vi "test_Are All Channels Defined.vi"(8 "error in":errorcluster) -> (0 "error out":errorcluster)   [LabVIEW 2020, in "Test_Routing Templates.lvlib"]
uses:
  Test_Routing Templates.lvlib
  Routing Channel Templates/Abstract Routing Channel Template/Abstract Routing Channel Template.lvclass/Abstract Routing Channel Template.ctl
  Routing Channel Templates/JSON Routing Channel Template/JSON Routing Channel Template.lvclass
  C:/Users/mjacobso/Desktop/SCM/Routing-Faulting/Source/Routing and Faulting/Routing Templates/Routing Channel Templates/Abstract Routing Channel Template/Abstract Routing Channel Template.lvclass
  <vilib>/addons/_JKI Toolkits/Caraya/classes/Assert/Assert False.vi
  <vilib>/addons/_JKI Toolkits/Caraya/classes/Assert/Assert True.vi
  <vilib>/addons/_JKI Toolkits/Caraya/classes/Test/Test.lvclass
  <vilib>/addons/_JKI Toolkits/Caraya/classes/Assert/Assert.lvclass
  Routing Channel Templates/Abstract Routing Channel Template/Abstract Routing Channel Template.lvclass
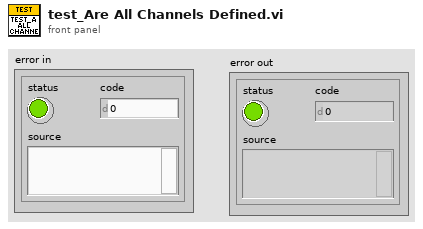
[diagram p1: front panel]
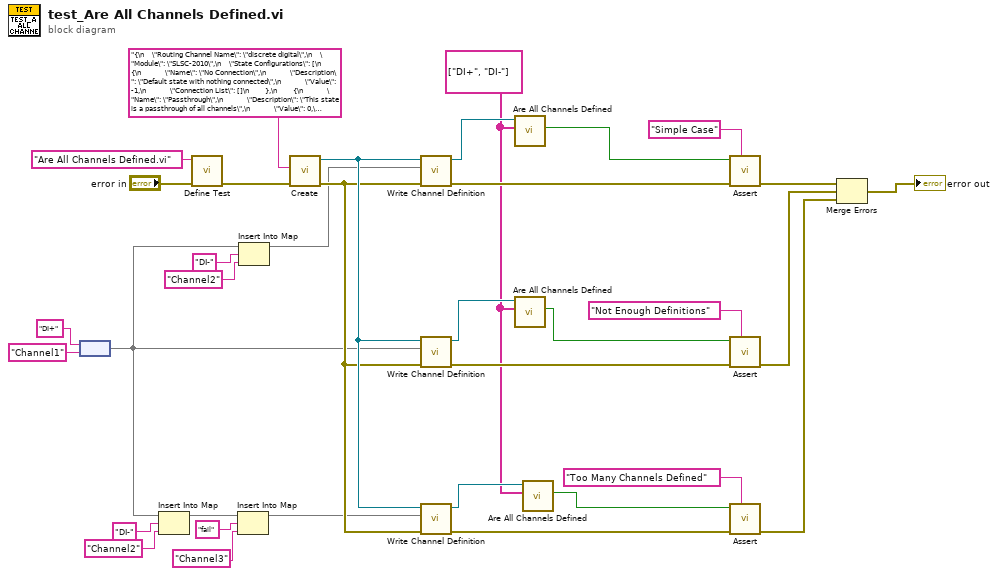
[diagram p0: block diagram]
diagram:
  w13 = string[] ["DI+", "DI-"]
  n1 = node ("Build Map")("DI+", "Channel1") -> (w5:map{string, string})
  n2 = Insert Into Map(map in=w5, key="DI-", value="Channel2") -> (map out=w4:map{string, string})  [unwired: 2 out]
  n3 = call <vilib>:"Define Test.vi"("error in (no error)"="error in", "Label (VI Title)"="Are All Channels Defined.vi") -> ("error out"=w33:errorcluster)  [unwired: 9 in]
  n4 = Insert Into Map(map in=w4, key="fail", value="Channel3") -> (map out=w1:map{string, string})  [unwired: 2 out]
  n5 = Insert Into Map(map in=w5, key="DI-", value="Channel2") -> (map out=w8:map{string, string})  [unwired: 2 out]
  n6 = call "Create.vi"("error in (no error)"=w33, "JSON"="{\n    \"Routing Channel Name\": \"discrete digital\",\n    \"Module\": \"SLSC-2010\",\n    \"State Configurations\": [\n        {\n            \"Name\": \"No Connection\",\n            \"Description\": \"Default state with nothing connected\",\n            \"Value\": -1,\n            \"Connection List\": []\n        },\n        {\n            \"Name\": \"Passthrough\",\n            \"Description\": \"This state is a passthrough of all channels\",\n            \"Value\": 0,\n            \"Connection List\": [\n                {\n                    \"Channel\": \"DI+\",\n                    \"Connection Type\": \"Passthrough\"\n                },\n                {\n                    \"Channel\": \"DI-\",\n                    \"Connection Type\": \"Passthrough\"\n                }\n            ]\n        },\n        {\n            \"Name\": \"Real-Sim\",\n            \"Description\": \"Connect J1 to J2 pins\",\n            \"Value\": 1,\n            \"Connection List\": [\n                {\n                    \"Channel\": \"DI+\",\n                    \"Connection Type\": \"Real-Sim\"\n                },\n                {\n                    \"Channel\": \"DI-\",\n                    \"Connection Type\": \"Real-Sim\"\n                }\n            ]\n        }\n    ]\n}" ("text")) -> ("error out"=w25:errorcluster, "JSON Routing Channel Template out"=w26:refnum<class "JSON Routing Channel Template.lvclass">)  [unwired: 8 in]
  n7 = call "Write Channel Definition.vi"("error in (no error)"=w25, "Channel Definition"=w8, "Abstract Routing Channel Template in"=w26) -> ("error out"=w19:errorcluster, "Abstract Routing Channel Template out"=w15:refnum<class "JSON Routing Channel Template.lvclass">)  [unwired: 7 in]
  n8 = call "Write Channel Definition.vi"("error in (no error)"=w25, "Channel Definition"=w5, "Abstract Routing Channel Template in"=w26) -> ("error out"=w28:errorcluster, "Abstract Routing Channel Template out"=w23:refnum<class "JSON Routing Channel Template.lvclass">)  [unwired: 7 in]
  n9 = call "Write Channel Definition.vi"("error in (no error)"=w25, "Channel Definition"=w1, "Abstract Routing Channel Template in"=w26) -> ("error out"=w27:errorcluster, "Abstract Routing Channel Template out"=w24:refnum<class "JSON Routing Channel Template.lvclass">)  [unwired: 7 in]
  n10 = call "Are All Channels Defined.vi"("Channels"=w13, "JSON RCT"=w15) -> ("All Defined?"=w31:bool)  [unwired: 8 in, 1 out]
  n11 = call "Are All Channels Defined.vi"("Channels"=w13, "JSON RCT"=w23) -> ("All Defined?"=w22:bool)  [unwired: 8 in, 1 out]
  n12 = call "Are All Channels Defined.vi"("Channels"=w13, "JSON RCT"=w24) -> ("All Defined?"=w21:bool)  [unwired: 8 in, 1 out]
  n13 = call-poly <vilib>:"Assert.vi"("Label"="Simple Case", "error in (no error)"=w19, "True?"=w31) -> ("error out"=w32:errorcluster)  [unwired: 8 in]
  n14 = call-poly <vilib>:"Assert.vi"("Label"="Not Enough Definitions", "error in (no error)"=w28, "False?"=w22) -> ("error out"=w17:errorcluster)  [unwired: 8 in]
  n15 = call-poly <vilib>:"Assert.vi"("Label"="Too Many Channels Defined", "error in (no error)"=w27, "True?"=w21) -> ("error out"=w16:errorcluster)  [unwired: 8 in]
  n16 = Merge Errors(w32, w17, w16) -> (→"error out":errorcluster)
